vi "xtime.vi"(11 "Numeric in":u8 format="%.0x") -> (3 "Numeric out":u8 format="%.0x")   [LabVIEW 2017]
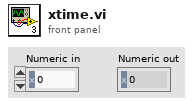
[diagram p1: front panel]
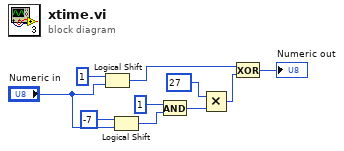
[diagram p0: block diagram]
diagram:
  n1 = Logical Shift(y=i16 1, x="Numeric in") -> (x << y=w9:u8)
  n2 = Logical Shift(y=i16 -7, x="Numeric in") -> (x << y=w4:u8)
  n3 = And(x=u8 1, y=w4) -> (x .and. y?=w6:u8)
  n4 = Multiply(x=u8 27, y=w6) -> (x*y=w8:u8)
  n5 = Exclusive Or(1:w8, 2:w9) -> (0:→"Numeric out":u8)
